vi "ID Pool.Create.vi"(7 "FIFO Debug Flags":refnum<class "FIFO Flags.lvclass">, 8 "error in (no error)":errorcluster, 10 "number of IDs":u32, 11 "ID Pool type":refnum<class "ID Pool.lvclass">) -> (0 "error out":errorcluster, 3 "ID Pool out":refnum<class "ID Pool.lvclass">)   [LabVIEW 2017, in "DSF Core.lvlib" / "ID Pool.lvclass"]
uses:
  ID Pool.lvclass
  C:/Git/DSF/dsf core/Source/Engine/Classes/Thread Pool/Pool.lvclass
  Debug/FIFO Flags.lvclass
  Pool.lvclass/Pool.ctl
  Debug/FIFO Flags.lvclass/FIFO Flags.ctl
  Pool.Get FIFO.vi
  Pool.Get Debug Flags.vi
  Debug/FIFO Flags.Get Infinite Timeouts.vi
  Pool.lvclass
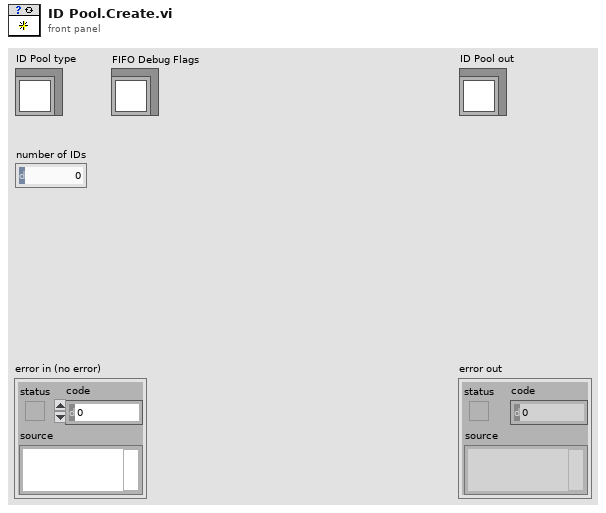
[diagram p1: front panel]
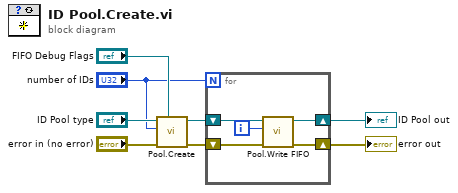
[diagram p0: block diagram]
diagram:
  n1 = call "Pool.Create.vi"("FIFO Debug Flags"="FIFO Debug Flags", "error in (no error)"="error in (no error)", "number of elements"="number of IDs", "Pool type"="ID Pool type") -> ("error out"=w3:errorcluster, "Pool"=w4:refnum<class "ID Pool.lvclass">)  [unwired: 6 in]
  n2 = for {
    N: "number of IDs" -> [_]
    shift-right: [w11] -> w8
    shift-left: w4 -> [w13]
    shift-right: [w10] -> w7
    shift-left: w3 -> [w12]
    i -> [w9]
    n3 = call "Pool.Write FIFO.vi"("error in (no error)"=w12, "element"=w9, "Pool in"=w13) -> ("error out"=w10:errorcluster, "Pool out"=w11:refnum<class "ID Pool.lvclass">)  [unwired: 6 in, 1 out]
  }
  "error out" <- w7
  "ID Pool out" <- w8
